vi "Write Home Params Cluster.vi"(8 "error in (no error)":errorcluster, 10 "Home Params Cluster":T1={"Home Mode"=enum."EZ+EL", "Home Dir"=enum."positive+", "Home Pos Shift"=0.0}, 11 "Motor Configuration in":refnum<class "Motor Configuration.lvclass">) -> (0 "error out":errorcluster, 3 "Motor Configuration out":refnum<class "Motor Configuration.lvclass">)   [LabVIEW 2016, in "Hardware.lvlib" / "Motor.lvlib" / "Motor Configuration.lvclass"]
uses:
  <userlib>/Common Components/Hardware/Motor/Motor Config/Motor Configuration.lvclass
  <userlib>/Common Components/Hardware/Motor/Motor/Home Params.ctl
  <userlib>/Common Components/Hardware/Motor/Motor/Home Mode.ctl
  <userlib>/Common Components/Hardware/Motor/Motor/Home Dir.ctl
  <userlib>/Common Components/Hardware/Motor/Motor/Motor.lvclass/Motor.ctl
  <userlib>/Common Components/Hardware/Motor/Motor Config/Accessors/Read Motor Obj.vi
  <userlib>/Common Components/Hardware/Motor/Motor Config/Accessors/Write Motor Obj.vi
  <userlib>/Common Components/Hardware/Motor/Motor/Motor.lvclass
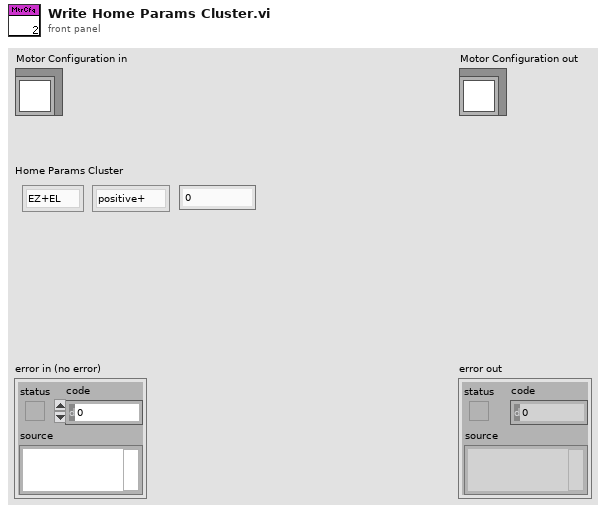
[diagram p1: front panel]
types:
  T1 = typedef "Hardware.lvlib/Motor.lvlib/Motor.lvclass/Home Params.ctl" = cluster{"Home Mode":T2, "Home Dir":T3, "Home Pos Shift":dbl}
  T2 = typedef "Hardware.lvlib/Motor.lvlib/Motor.lvclass/Home Mode.ctl" = enum16{"EZ+EL", "EZ only"}
  T3 = typedef "Hardware.lvlib/Motor.lvlib/Motor.lvclass/Home Dir.ctl" = enum16{"negative-", "positive+"}
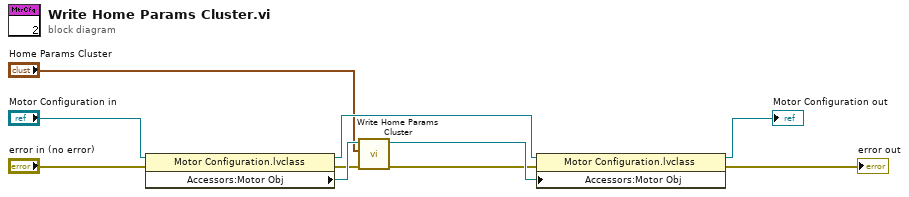
[diagram p0: block diagram]
diagram:
  n1 = property class="Motor Configuration.lvclass"(reference="Motor Configuration in", error in="error in (no error)") -> (reference out=w10:refnum<class "Motor Configuration.lvclass">, error out=w7:errorcluster, "Accessors:Motor Obj"=w9:refnum<class "Motor.lvclass">)
  n2 = call <userlib>:"Write Home Params Cluster.vi"("error in (no error)"=w7, "Home Params Cluster"="Home Params Cluster", "Motor in"=w9) -> ("error out"=w6:errorcluster, "Motor out"=w8:refnum<class "Motor.lvclass">)  [unwired: 7 in]
  n3 = property class="Motor Configuration.lvclass"(reference=w10, error in=w6, "Accessors:Motor Obj"=w8) -> (reference out=→"Motor Configuration out":refnum<class "Motor Configuration.lvclass">, error out=→"error out":errorcluster)
